vi "daq init all.vi"(6 "error in":errorcluster, 8 "rate 2":dbl=25000.0 format="%0.2f", 9 "number of samples 2":i32=25000, 10 "rate":dbl=25000.0 format="%0.2f", 11 "number of samples":i32=25000) -> (0 "error out":errorcluster, 3 "output cluster":T1)   [LabVIEW 2013]
uses:
  <vilib>/DAQmx/configure/timing.llb/DAQmx Timing (Sample Clock).vi
  <vilib>/DAQmx/create/channels.llb/DAQmx Create Channel (AI-Voltage-Basic).vi
  <vilib>/DAQmx/create/channels.llb/DAQmx Create Channel (TEDS-AI-Voltage-Basic).vi
  <vilib>/DAQmx/create/scale.llb/DAQmx Create Scale (Linear).vi
  <vilib>/DAQmx/create/channels.llb/DAQmx Create Channel (TEDS-AI-Current-Basic).vi
  <vilib>/DAQmx/create/channels.llb/DAQmx Create Channel (AI-Current-Basic).vi
  <resource>/objmgr/daqmx.rc
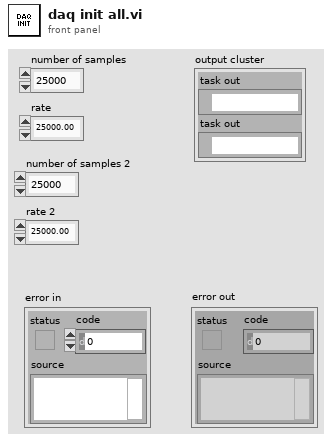
[diagram p1: front panel]
types:
  T1 = cluster{"task out":refnum<k21>, "task out":refnum<k21>}
  T2 = cluster{"name":string, "slope":dbl, "y-intercept":dbl, "pre-scaled units":i32, "scaled units":string}[]
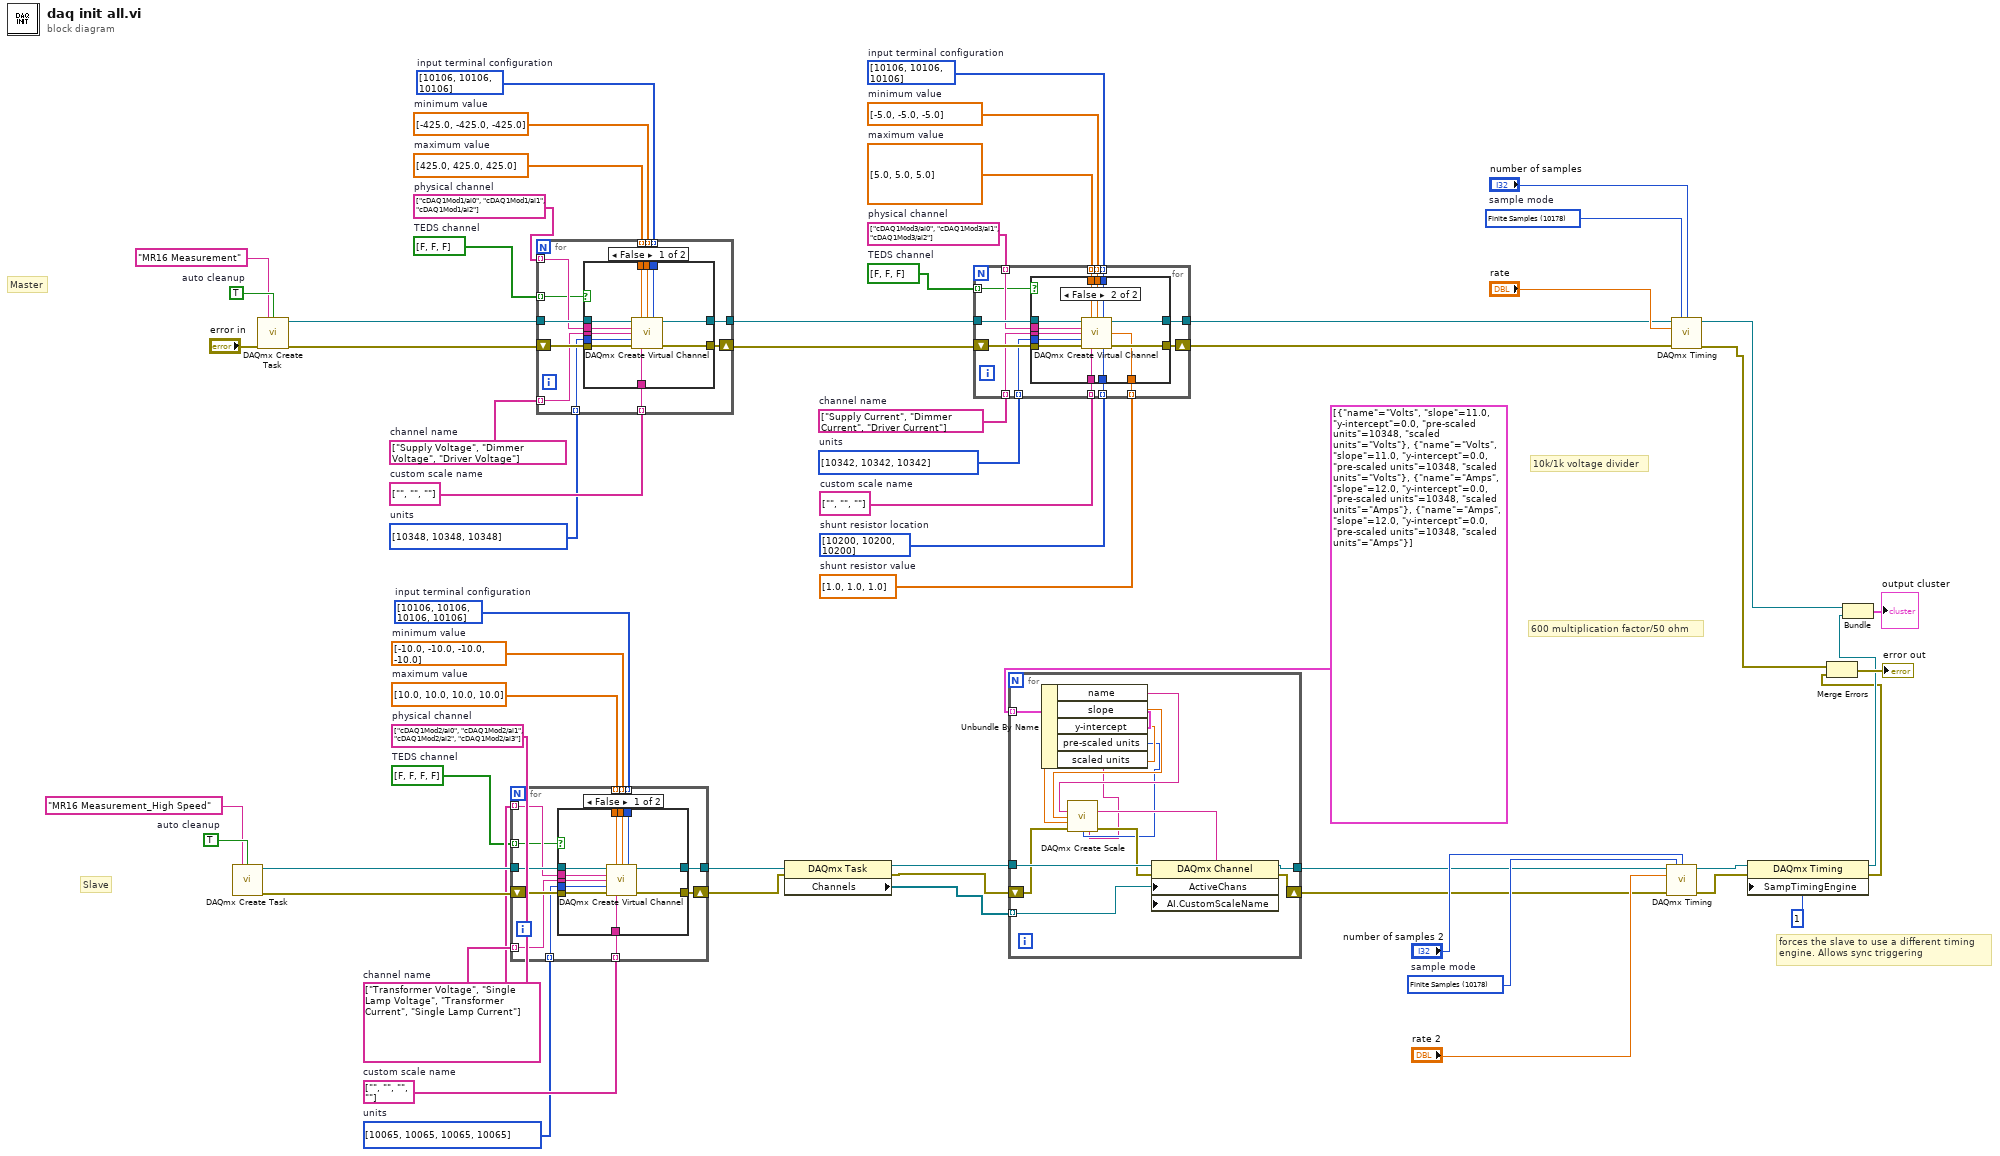
[diagram p0: block diagram]
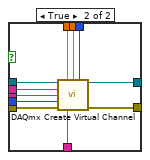
[diagram p2: hidden frame]
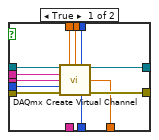
[diagram p3: hidden frame]
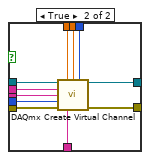
[diagram p4: hidden frame]
diagram:
  w19 = 10178 items=["Finite Samples"=10178, "Continuous Samples"=10123, "Hardware Timed Single Point"=12522]  # sample mode
  w22 = bool[] [FALSE, FALSE, FALSE, FALSE]  # TEDS channel
  w26 = string[] ["", "", "", ""]  # custom scale name
  w25 = i32[] [10065, 10065, 10065, 10065] items=["Volts"=10348, "From TEDS"=12516, "From Custom Scale"=10065]  # units
  w24 = string[] ["Transformer Voltage", "Single Lamp Voltage", "Transformer Current", "Single Lamp Current"]  # channel name
  w23 = string[] ["cDAQ1Mod2/ai0", "cDAQ1Mod2/ai1", "cDAQ1Mod2/ai2", "cDAQ1Mod2/ai3"]  # physical channel
  w27 = dbl[] [10.0, 10.0, 10.0, 10.0]  # maximum value
  w28 = dbl[] [-10.0, -10.0, -10.0, -10.0]  # minimum value
  w29 = i32[] [10106, 10106, 10106, 10106] items=["default"=-1, "RSE"=10083, "NRSE"=10078, "Differential"=10106, "Pseudodifferential"=12529]  # input terminal configuration
  w31 = TRUE  # auto cleanup
  w35 = string[] ["", "", ""]  # custom scale name
  w37 = 10178 items=["Finite Samples"=10178, "Continuous Samples"=10123, "Hardware Timed Single Point"=12522]  # sample mode
  w40 = bool[] [FALSE, FALSE, FALSE]  # TEDS channel
  w42 = i32[] [10200, 10200, 10200] items=["Internal"=10200, "External"=10167]  # shunt resistor location
  w41 = dbl[] [1.0, 1.0, 1.0]  # shunt resistor value
  w45 = i32[] [10342, 10342, 10342] items=["Amps"=10342, "From TEDS"=12516, "From Custom Scale"=10065]  # units
  w44 = string[] ["Supply Current", "Dimmer Current", "Driver Current"]  # channel name
  w43 = string[] ["cDAQ1Mod3/ai0", "cDAQ1Mod3/ai1", "cDAQ1Mod3/ai2"]  # physical channel
  w46 = dbl[] [5.0, 5.0, 5.0]  # maximum value
  w47 = dbl[] [-5.0, -5.0, -5.0]  # minimum value
  w48 = i32[] [10106, 10106, 10106] items=["default"=-1, "RSE"=10083, "NRSE"=10078, "Differential"=10106, "Pseudodifferential"=12529]  # input terminal configuration
  w50 = bool[] [FALSE, FALSE, FALSE]  # TEDS channel
  w55 = string[] ["", "", ""]  # custom scale name
  w54 = i32[] [10348, 10348, 10348] items=["Volts"=10348, "From TEDS"=12516, "From Custom Scale"=10065]  # units
  w53 = string[] ["Supply Voltage", "Dimmer Voltage", "Driver Voltage"]  # channel name
  w52 = string[] ["cDAQ1Mod1/ai0", "cDAQ1Mod1/ai1", "cDAQ1Mod1/ai2"]  # physical channel
  w56 = dbl[] [425.0, 425.0, 425.0]  # maximum value
  w57 = dbl[] [-425.0, -425.0, -425.0]  # minimum value
  w58 = i32[] [10106, 10106, 10106] items=["default"=-1, "RSE"=10083, "NRSE"=10078, "Differential"=10106, "Pseudodifferential"=12529]  # input terminal configuration
  w60 = TRUE  # auto cleanup
  # "10k/1k voltage divider"
  # "600 multiplication factor/50 ohm"
  # "forces the slave to use a different timing \nengine. Allows sync triggering"
  # "Slave"
  # "Master"
  n1 = call <vilib>:"DAQmx Create Task.vi"("new task name"="MR16 Measurement_High Speed", "auto cleanup"=w31) -> ("task out"=w30:refnum<k21>, "error out"=w32:errorcluster)  [unwired: 12 in]
  n2 = call <vilib>:"DAQmx Create Task.vi"("new task name"="MR16 Measurement", "auto cleanup"=w60, "error in"="error in") -> ("task out"=w59:refnum<k21>, "error out"=w61:errorcluster)  [unwired: 11 in]
  n3 = for {
    tunnel: w30 -> [w71]
    tunnel: w29 -> [w72] mode=indexing
    tunnel: w28 -> [w73] mode=indexing
    tunnel: w27 -> [w74] mode=indexing
    tunnel: w26 -> [w64] mode=indexing
    tunnel: w25 -> [w65] mode=indexing
    tunnel: w24 -> [w67] mode=indexing
    tunnel: w23 -> [w66] mode=indexing
    tunnel: [w69] -> w15
    shift-right: [w68] -> w14
    shift-left: w32 -> [w70]
    tunnel: w22 -> [w63] mode=indexing
    n4 = case shown="False" w63 {
      tunnel: w74 -> [w85 w90]
      tunnel: w73 -> [w84 w91]
      tunnel: w72 -> [w83 w92]
      tunnel: w71 -> [w82 w96]
      tunnel: w70 -> [w81 w95]
      tunnel: [w80 w93] -> w69
      tunnel: [w79 w94] -> w68
      tunnel: w67 -> [w78 w88]
      tunnel: w66 -> [w77 w89]
      tunnel: w65 -> [w76 w87]
      tunnel: w64 -> [w75 w86]
      frame False {
        n5 = call-poly <vilib>:"DAQmx Create Virtual Channel.vi"("task in"=w82, "maximum value"=w85, "minimum value"=w84, "input terminal configuration"=w83, "physical channels"=w77, "name to assign"=w78, "units"=w76, "error in"=w81, "custom scale name"=w75) -> ("task out"=w80:refnum<k21>, "error out"=w79:errorcluster)  [unwired: 5 in]
      }
      frame True {
        n6 = call-poly <vilib>:"DAQmx Create Virtual Channel.vi"("task in"=w96, "maximum value"=w90, "minimum value"=w91, "input terminal configuration"=w92, "physical channels"=w89, "name to assign"=w88, "units"=w87, "error in"=w95, "custom scale name"=w86) -> ("task out"=w93:refnum<k21>, "error out"=w94:errorcluster)  [unwired: 5 in]
      }
    }
  }
  n7 = for {
    tunnel: w59 -> [w105]
    tunnel: w58 -> [w106] mode=indexing
    tunnel: w57 -> [w107] mode=indexing
    tunnel: w56 -> [w108] mode=indexing
    tunnel: w55 -> [w98] mode=indexing
    tunnel: w54 -> [w99] mode=indexing
    tunnel: w53 -> [w101] mode=indexing
    tunnel: w52 -> [w100] mode=indexing
    tunnel: [w103] -> w49
    shift-right: [w102] -> w51
    shift-left: w61 -> [w104]
    tunnel: w50 -> [w97] mode=indexing
    n8 = case shown="False" w97 {
      tunnel: w108 -> [w119 w124]
      tunnel: w107 -> [w118 w125]
      tunnel: w106 -> [w117 w126]
      tunnel: w105 -> [w116 w130]
      tunnel: w104 -> [w115 w129]
      tunnel: [w114 w127] -> w103
      tunnel: [w113 w128] -> w102
      tunnel: w101 -> [w112 w122]
      tunnel: w100 -> [w111 w123]
      tunnel: w99 -> [w110 w121]
      tunnel: w98 -> [w109 w120]
      frame False {
        n9 = call-poly <vilib>:"DAQmx Create Virtual Channel.vi"("task in"=w116, "maximum value"=w119, "minimum value"=w118, "input terminal configuration"=w117, "physical channels"=w111, "name to assign"=w112, "units"=w110, "error in"=w115, "custom scale name"=w109) -> ("task out"=w114:refnum<k21>, "error out"=w113:errorcluster)  [unwired: 5 in]
      }
      frame True {
        n10 = call-poly <vilib>:"DAQmx Create Virtual Channel.vi"("task in"=w130, "maximum value"=w124, "minimum value"=w125, "input terminal configuration"=w126, "physical channels"=w123, "name to assign"=w122, "units"=w121, "error in"=w129, "custom scale name"=w120) -> ("task out"=w127:refnum<k21>, "error out"=w128:errorcluster)  [unwired: 5 in]
      }
    }
  }
  n11 = property class="DAQmx Task"(reference=w15, error in=w14) -> (reference out=w13:refnum<k21>, error out=w12:errorcluster, "Channels"=w10:refnum<k21>[])
  n12 = for {
    tunnel: w49 -> [w141]
    tunnel: w48 -> [w144] mode=indexing
    tunnel: w47 -> [w143] mode=indexing
    tunnel: w46 -> [w142] mode=indexing
    tunnel: w45 -> [w135] mode=indexing
    tunnel: w44 -> [w137] mode=indexing
    tunnel: w43 -> [w136] mode=indexing
    tunnel: [w139] -> w34
    tunnel: w42 -> [w134] mode=indexing
    tunnel: w41 -> [w133] mode=indexing
    shift-right: [w138] -> w33
    shift-left: w51 -> [w140]
    tunnel: w40 -> [w132] mode=indexing
    tunnel: w35 -> [w131] mode=indexing
    n13 = case shown="False" w132 {
      tunnel: w144 -> [w156 w169]
      tunnel: w143 -> [w155 w168]
      tunnel: w142 -> [w154 w167]
      tunnel: w141 -> [w153 w166]
      tunnel: w140 -> [w152 w165]
      tunnel: [w151 w164] -> w139
      tunnel: [w150 w163] -> w138
      tunnel: w137 -> [w149 w162]
      tunnel: w136 -> [w148 w161]
      tunnel: w135 -> [w147 w160]
      tunnel: w134 -> [w146 w159]
      tunnel: w133 -> [w145 w158]
      tunnel: w131 -> [_ w157]
      frame True {
        n14 = call-poly <vilib>:"DAQmx Create Virtual Channel.vi"("task in"=w153, "maximum value"=w154, "minimum value"=w155, "input terminal configuration"=w156, "physical channels"=w148, "name to assign"=w149, "external shunt resistor value"=w145, "units"=w147, "error in"=w152, "shunt resistor location"=w146) -> ("task out"=w151:refnum<k21>, "error out"=w150:errorcluster)  [unwired: 4 in]
      }
      frame False {
        n15 = call-poly <vilib>:"DAQmx Create Virtual Channel.vi"("task in"=w166, "maximum value"=w167, "minimum value"=w168, "input terminal configuration"=w169, "physical channels"=w161, "name to assign"=w162, "external shunt resistor value"=w158, "units"=w160, "error in"=w165, "custom scale name"=w157, "shunt resistor location"=w159) -> ("task out"=w164:refnum<k21>, "error out"=w163:errorcluster)  [unwired: 3 in]
      }
    }
  }
  n16 = for {
    tunnel: w13 -> [w182]
    tunnel: [w181] -> w17
    tunnel: w10 -> [w177] mode=indexing
    shift-right: [w180] -> w16
    shift-left: w12 -> [w176]
    tunnel: T2 [{"name"="Volts", "slope"=11.0, "y-intercept"=0.0, "pre-scaled units"=10348, "scaled units"="Volts"}, {"name"="Volts", "slope"=11.0, "y-intercept"=0.0, "pre-scaled units"=10348, "scaled units"="Volts"}, {"name"="Amps", "slope"=12.0, "y-intercept"=0.0, "pre-scaled units"=10348, "scaled units"="Amps"}, {"name"="Amps", "slope"=12.0, "y-intercept"=0.0, "pre-scaled units"=10348, "scaled units"="Amps"}] -> [w175] mode=indexing
    n17 = Unbundle By Name(w175) -> ("name"=w172:string, "slope"=w173:dbl, "y-intercept"=w174:dbl, "pre-scaled units"=w171:i32, "scaled units"=w170:string)
    n18 = call-poly <vilib>:"DAQmx Create Scale.vi"("name"=w172, "slope"=w173, "y-intercept"=w174, "error in"=w176, "pre-scaled units"=w171, "scaled units"=w170) -> ("scale out"=w179:tag, "error out"=w178:errorcluster)  [unwired: 8 in]
    n19 = property class="DAQmx Channel"(reference=w182, error in=w178, "ActiveChans"=w177, "AI.CustomScaleName"=w179) -> (reference out=w181:refnum<k21>, error out=w180:errorcluster)
  }
  n20 = call-poly <vilib>:"DAQmx Timing.vi"("task/channels in"=w17, "sample mode"=w19, "samples per channel"="number of samples 2", "rate"="rate 2", "error in"=w16) -> ("task out"=w6:refnum<k21>, "error out"=w5:errorcluster)  [unwired: 9 in]
  n21 = call-poly <vilib>:"DAQmx Timing.vi"("task/channels in"=w34, "sample mode"=w37, "samples per channel"="number of samples", "rate"="rate", "error in"=w33) -> ("task out"=w9:refnum<k21>, "error out"=w7:errorcluster)  [unwired: 9 in]
  n22 = property class="DAQmx Timing"(reference=w6, error in=w5, "SampTimingEngine"=u32 1) -> (reference out=w4:refnum<k21>, error out=w3:errorcluster)
  n23 = Merge Errors(w7, w3) -> (→"error out":errorcluster)
  n24 = Bundle("task out"=w9, "task out"=w4) -> (→"output cluster":T1)  [unwired: 1 in]
